vi "Get Variant Data Type.vi"(11 "variant":variant) -> (3 "Data Type":string[](array[string]))   [LabVIEW 2014]
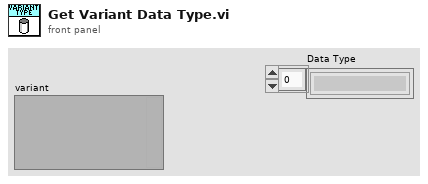
[diagram p1: front panel]
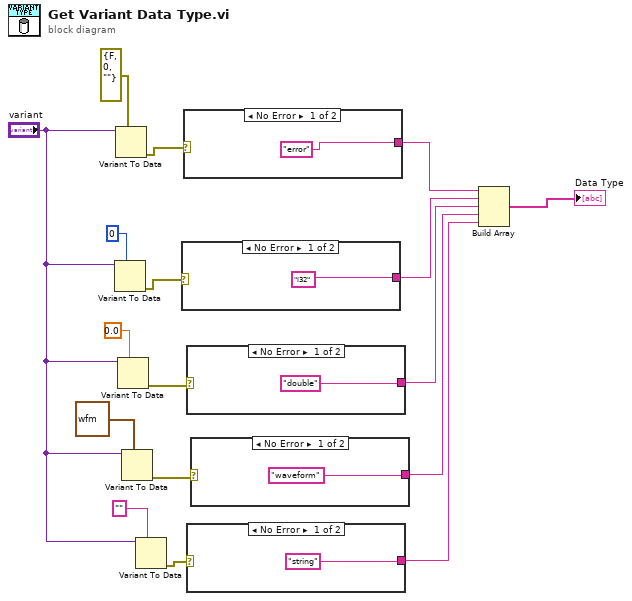
[diagram p0: block diagram]
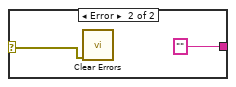
[diagram p2: hidden frame]
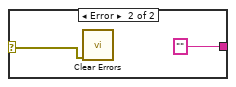
[diagram p3: hidden frame]
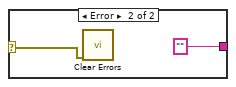
[diagram p4: hidden frame]
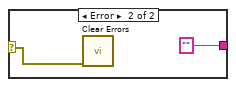
[diagram p5: hidden frame]
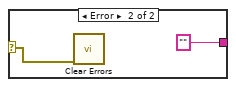
[diagram p6: hidden frame]
diagram:
  n1 = Variant To Data(type=0, Variant="variant") -> (error out=w14:errorcluster)  [unwired: 1 in, 1 out]
  n2 = Variant To Data(type=errorcluster {"status"=FALSE, "code"=0, "source"=""} ("error constant"), Variant="variant") -> (error out=w17:errorcluster)  [unwired: 1 in, 1 out]
  n3 = Variant To Data(type=0.0, Variant="variant") -> (error out=w12:errorcluster)  [unwired: 1 in, 1 out]
  n4 = Variant To Data(type=waveform(dbl) {"t0"=timestamp(0 s since 1904-01-01), "dt"=1.0, "Y"=[]} ("Waveform"), Variant="variant") -> (error out=w7:errorcluster)  [unwired: 1 in, 1 out]
  n5 = Variant To Data(type="" ("Data Type"), Variant="variant") -> (error out=w4:errorcluster)  [unwired: 1 in, 1 out]
  n6 = case shown="No Error" w14 {
    selector: w14 -> [_ w20]
    tunnel: ["i32" ("Data Type") "" ("Data Type")] -> w10
    frame No Error {
    }
    frame Error {
      n7 = call <vilib>:"Clear Errors.vi"("error in (no error)"=w20) -> ()  [unwired: 5 in, 2 out]
    }
  }
  n8 = case shown="No Error" w17 {
    selector: w17 -> [_ w23]
    tunnel: ["error" ("Data Type") "" ("Data Type")] -> w11
    frame No Error {
    }
    frame Error {
      n9 = call <vilib>:"Clear Errors.vi"("error in (no error)"=w23) -> ()  [unwired: 5 in, 2 out]
    }
  }
  n10 = case shown="No Error" w12 {
    selector: w12 -> [_ w26]
    tunnel: ["double" ("Data Type") "" ("Data Type")] -> w9
    frame No Error {
    }
    frame Error {
      n11 = call <vilib>:"Clear Errors.vi"("error in (no error)"=w26) -> ()  [unwired: 5 in, 2 out]
    }
  }
  n12 = case shown="No Error" w4 {
    selector: w4 -> [_ w29]
    tunnel: ["string" ("Data Type") "" ("Data Type")] -> w1
    frame No Error {
    }
    frame Error {
      n13 = call <vilib>:"Clear Errors.vi"("error in (no error)"=w29) -> ()  [unwired: 5 in, 2 out]
    }
  }
  n14 = case shown="No Error" w7 {
    selector: w7 -> [_ w32]
    tunnel: ["waveform" ("Data Type") "" ("Data Type")] -> w5
    frame No Error {
    }
    frame Error {
      n15 = call <vilib>:"Clear Errors.vi"("error in (no error)"=w32) -> ()  [unwired: 5 in, 2 out]
    }
  }
  n16 = Build Array(w11, w10, w9, w5, w1) -> (→"Data Type":string[])
